vi "Read Multiple Event Registration.vi"(6 "number of event structures":u16=2, 10 "channel":T1) -> (2 "event registration refnums":refnum<event-registration>[](array[refnum]))   [LabVIEW 2019, in "Cmd-Data Event Messenger.lvlib"]
doc: "<p>Reads multiple <a href=\"nihelplauncher://docs/csh?context=lvcore_lvconcepts_using_events_in_labview\">event registration</a> refnums for an Event Messenger <a href=\"nihelplauncher://docs/csh?context=lvcore_lvconcepts_channel_wires_intro\">channel</a> and makes the refnums available to one or more <a href=\"nihelplauncher://docs/csh?context=lvcore_glang_event_structure\">Event structures</a>.</p>"
uses:
  Cmd-Data Event Messenger.lvlib
  <resource>/ChannelSupport/_ChannelSupport/GetErrors/FpgaChannelWireNotSupported.xnode
  ChannelOp.ctl
  ))Channel.ctl
  Event Data.ctl
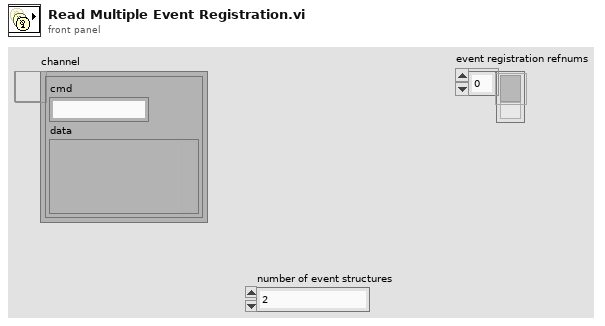
[diagram p1: front panel]
types:
  T1 = typedef "Cmd-Data Event Messenger.lvlib/))Channel.ctl" = refnum<queue>
  T2 = typedef "Cmd-Data Event Messenger.lvlib/ChannelOp.ctl" = enum16{"init", "write", "register", "replicate", "probe"}
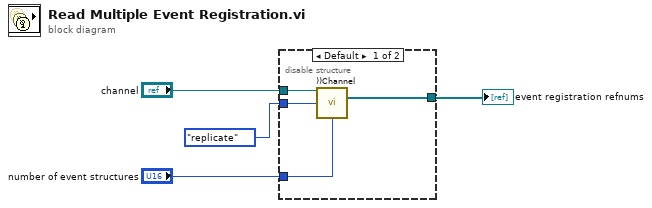
[diagram p0: block diagram]
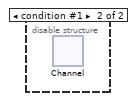
[diagram p2: hidden frame]
diagram:
  n1 = disable-structure shown="Default" {
    disable-tunnel: ChannelOp."replicate" ("channelOp") -> [w8 _]
    disable-tunnel: "channel" -> [w7 _]
    disable-tunnel: [w6 _] -> w1
    disable-tunnel: "number of event structures" -> [w5 _]
    frame condition #0 (active) {
      n2 = call "))Channel.vi"("channel in"=w7, "channelOp"=w8, "# event structures"=w5) -> ("event registration refnums"=w6:refnum<event-registration>[])  [unwired: 8 in, 4 out]
    }
    frame condition #1 {
      n3 = xnode "Channel"() -> ()
    }
  }
  "event registration refnums" <- w1
